vi "GetParam.vi"(8 "error in (no error)":errorcluster caption="entrée d'erreur (pas d'erreur)", 11 "PolynomialFeatures.lvclass":refnum<class "PolynomialFeatures.lvclass">) -> (0 "error out":errorcluster caption="sortie d'erreur", 2 "PolynomialFeatures":T1={"degre"=2, "interaction_only"=FALSE, "include_bias"=TRUE, "order"="C"}, 3 "PolynomialFeatures.lvclass":refnum<class "PolynomialFeatures.lvclass">)   [LabVIEW 2020, in "PolynomialFeatures.lvclass"]
doc: "Get Parameters"
uses:
  PolynomialFeatures.lvclass
  PolynomialFeatures.lvclass/PolynomialFeatures.ctl
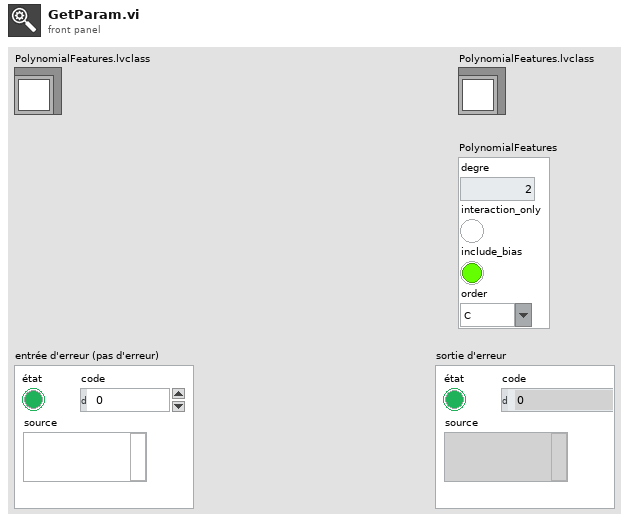
[diagram p1: front panel]
types:
  T1 = cluster{"degre":i32, "interaction_only":bool, "include_bias":bool, "order":string}
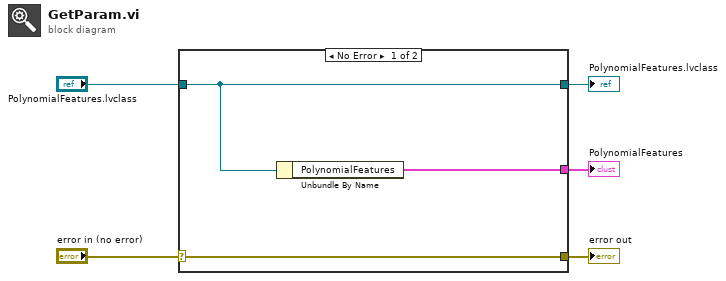
[diagram p0: block diagram]
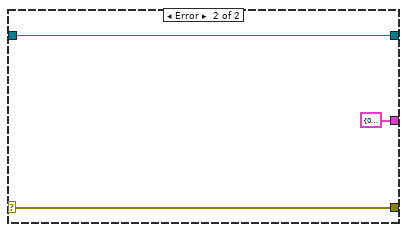
[diagram p2: hidden frame]
diagram:
  n1 = case shown="No Error" "error in (no error)" {
    selector: "error in (no error)" -> [w8 w10]
    tunnel: [w8 w10] -> w4
    tunnel: [w7 w11] -> w2
    tunnel: "PolynomialFeatures.lvclass" -> [w7 w11]
    tunnel: [w6 T1 {"degre"=0, "interaction_only"=FALSE, "include_bias"=FALSE, "order"=""} ("PolynomialFeatures")] -> w1
    frame No Error {
      n2 = Unbundle By Name(w7) -> ("PolynomialFeatures"=w6:T1)
    }
    frame Error {
    }
  }
  "error out" <- w4
  "PolynomialFeatures.lvclass" <- w2
  "PolynomialFeatures" <- w1
